vi "Write Person.vi"(10 "TRIARC_PROCESS":refnum<class "Person.lvclass">, 11 "Person Test in":refnum<class "Person Test.lvclass">) -> (3 "Person Test out":refnum<class "Person Test.lvclass">)   [LabVIEW 2020, in "Person Test.lvclass"]
uses:
  Person Test.lvclass
  Person Test.lvclass/Person Test.ctl
  Processes/People/Person/Person.lvclass
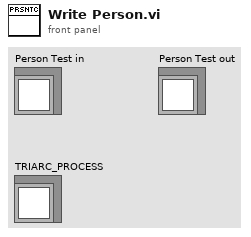
[diagram p1: front panel]
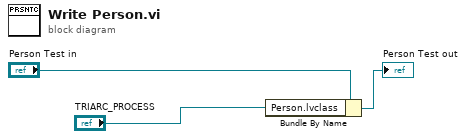
[diagram p0: block diagram]
diagram:
  n1 = Bundle By Name(cluster="Person Test in", "Person.lvclass"="TRIARC_PROCESS") -> (→"Person Test out":refnum<class "Person Test.lvclass">)
